vi "Array_Sensors.vi"(6 "error in 2":errorcluster, 7 "error in":errorcluster, 8 "Count":i32, 9 "Digital":refnum<k21>, 10 "Array":dbl[](array[numeric]), 11 "Analog":refnum<k21>) -> (0 "Iteración":i32, 1 "Voltage_in":dbl, 2 "Current":dbl, 3 "Watt":dbl, 4 "RPM":dbl, 5 "appended array":errorcluster[](array[cluster]))   [LabVIEW 2013, in "Test_Libraries.lvlib"]
uses:
  Proyecto/Test_Libraries.lvlib
  <vilib>/DAQmx/read.llb/DAQmx Read (Digital Bool 1Line 1Point).vi
  <vilib>/DAQmx/read.llb/DAQmx Read (Analog 2D DBL NChan NSamp).vi
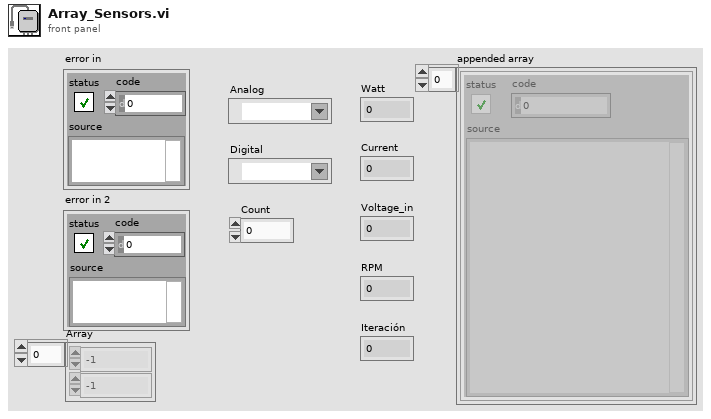
[diagram p1: front panel]
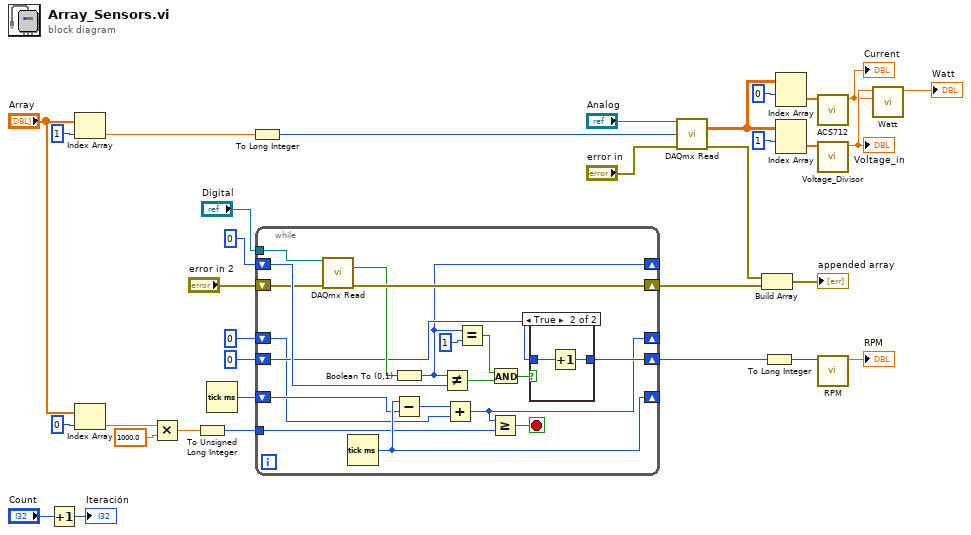
[diagram p0: block diagram]
diagram:
  n1 = Increment(x="Count") -> (x+1=→"Iteración":i32)
  n2 = Index Array(array="Array", index=1) -> (element=w7:dbl)
  n3 = Index Array(array="Array", index=0) -> (element=w4:dbl)
  n4 = Multiply(x=w4, y=1000.0) -> (x*y=w1:dbl)
  n5 = To Unsigned Long Integer(number=w1) -> (unsigned 32bit integer=w2:u32)
  n6 = Tick Count (ms)() -> (millisecond timer value=w12:u32)
  n7 = To Long Integer(number=w7) -> (32bit integer=w5:i32)
  n8 = while {
    tunnel: "Digital" -> [w51]
    shift-right: [w49] -> w16
    shift-left: "error in 2" -> [w50]
    shift-right: [w41] -> _
    shift-left: i16 0 -> [w52]
    shift-right: [w42] -> w10
    shift-left: 0 -> [w43]
    shift-right: [w40] -> _
    shift-left: w12 -> [w39]
    shift-right: [w36] -> _
    shift-left: u32 0 ("y") -> [w37]
    tunnel: w2 -> [w34]
    stop <- w35 stop-if-true
    n9 = call-poly <vilib>:"DAQmx Read.vi"("task/channels in"=w51, "error in"=w50) -> ("data"=w48:bool, "error out"=w49:errorcluster)  [unwired: 11 in, 1 out]
    n10 = Tick Count (ms)() -> (millisecond timer value=w40:u32)
    n11 = Boolean To (0,1)(Boolean=w48) -> (0, 1=w41:i16)
    n12 = Subtract(x=w40, y=w39) -> (x-y=w38:u32)
    n13 = Not Equal?(x=w41, y=w52) -> (x != y?=w45:bool)
    n14 = Add(x=w38, y=w37) -> (x+y=w36:u32)
    n15 = Equal?(x=w41, y=i16 1) -> (x = y?=w46:bool)
    n16 = Greater Or Equal?(x=w36, y=w34) -> (x >= y?=w35:bool)
    n17 = And(x=w46, y=w45) -> (x .and. y?=w44:bool)
    n18 = case shown="True" w44 {
      tunnel: w43 -> [w53 w54]
      tunnel: [w53 w55] -> w42
      frame False {
      }
      frame True {
        n19 = Increment(x=w54) -> (x+1=w55:i32)
      }
    }
  }
  n20 = call-poly <vilib>:"DAQmx Read.vi"("task/channels in"="Analog", "number of samples per channel"=w5, "error in"="error in") -> ("data"=w22:dbl[][], "error out"=w17:errorcluster)  [unwired: 10 in, 1 out]
  n21 = Build Array(w17, w16) -> (→"appended array":errorcluster[])
  n22 = To Long Integer(number=w10) -> (32bit integer=w20:i32)
  n23 = Index Array(array=w22, index (row)=0) -> (element=w24:dbl[])  [unwired: 1 in]
  n24 = Index Array(array=w22, index (row)=1) -> (element=w23:dbl[])  [unwired: 1 in]
  n25 = call "ACS712.vi"("ACS712"=w24) -> ("Current"=w31:dbl)  [unwired: 10 in]
  "Current" <- w31
  n26 = call "Voltage_Divisor.vi"("Voltage"=w23) -> ("Voltage_in"=w32:dbl)  [unwired: 10 in]
  "Voltage_in" <- w32
  n27 = call "RPM.vi"("Input"=w20) -> ("RPM"=→"RPM":dbl)  [unwired: 10 in]
  n28 = call "Watt.vi"("Current"=w31, "Voltage_in"=w32) -> ("Watt"=→"Watt":dbl)  [unwired: 9 in]
